vi "AK Namen.vi"(6 "Aktionen":T3, 7 "KV?":bool, 8 "EKFG Liste":string[](array[string]), 9 "AK Namen":string[](array[string]), 11 "Aktuelle Gasliste FT-IR":T1[](array[typedef])) -> (0 "EKFG Liste":string[](array[string]), 1 "AK Namen":string[](array[string]), 2 "Namen":string[](array[string]), 3 "AK Namen Liste":T2)   [LabVIEW 2020, in "AK-Schnittstelle.lvlib"]
uses:
  AK-Schnittstelle.lvlib
  AK Namen Aktionen.ctl
  AK Namen Listen.ctl
  Visualisierungs Elemente/String - Ausgabefeld.ctl
  SysLog/SysLog Interface.ctl
  Aktionen Gespeicherte Werte.ctl
  Allgemein/allgemeine Sub-VIs.lvlib
  Seiten/Gaszuordnung AO/Gaszuordnung AO.lvlib
  SysLog/SysLog.lvlib
  Aktion Array speichern.ctl
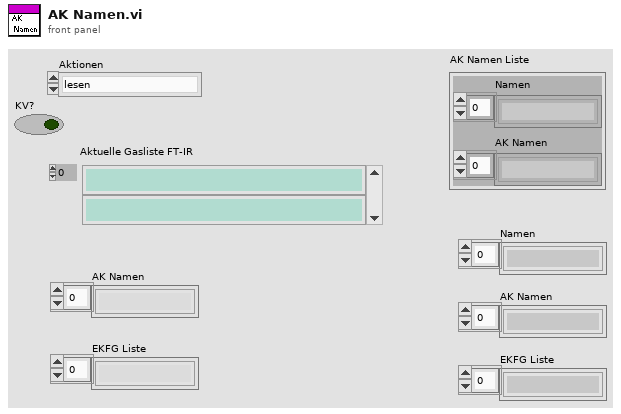
[diagram p1: front panel]
types:
  T1 = typedef "String - Ausgabefeld.ctl" = string
  T2 = typedef "AK-Schnittstelle.lvlib/AK Namen Listen.ctl" = cluster{"Namen":string[], "AK Namen":string[]}
  T3 = typedef "AK-Schnittstelle.lvlib/AK Namen Aktionen.ctl" = enum16{"lesen", "laden", "speichern Namen", "AK Namen", "Liste erstellen", "EKFG erstellen", "speichern EKFG", "EKFG schreiben", "Neuen Eintrag erzeugen"}
  T4 = typedef "SysLog.lvlib/SysLog Interface.ctl" = cluster{"FehlermeldungsCode":i32, "ErfolgsmeldungsCode":i32, "ParameterListenString":string, "Anzeige":bool, "SysLogIcon":enum16{"OK", "Warnung", "Fehler"}, "intern":bool}
  T5 = enum16{"open", "replace", "create", "open or create", "replace or create", "replace or create with confirmation"}
  T6 = typedef "AK-Schnittstelle.lvlib/Aktionen Gespeicherte Werte.ctl" = enum16{"lesen", "laden", "speichern", "Seriell", "TCP", "Diverse", "AKTIV", "AK-Namen"}
  T7 = typedef "AK-Schnittstelle.lvlib/Aktion Array speichern.ctl" = enum16{"AK Name ersetzen", "EKFG ersetzen", "Rezept fehler", "neues Rezept erstellen"}
  T8 = typedef "AK-Schnittstelle.lvlib/Diverse gespeicherte Werte.ctl" = cluster{"Kalibriergaseingang":i16, "SamplePoint":i16, "CalGas zu PNS":i16, "Gas-Reihenfolge":i16[], "Zeit 0-Gas":sgl, "Zeit CalGas":sgl, "AK Befehlssatz":T9}
  T9 = typedef "AK-Schnittstelle.lvlib/AK Befehlssatz.ctl" = enum16{"MEXA", "IAG v1.4", "AVL (Puma)", "PEUS"}
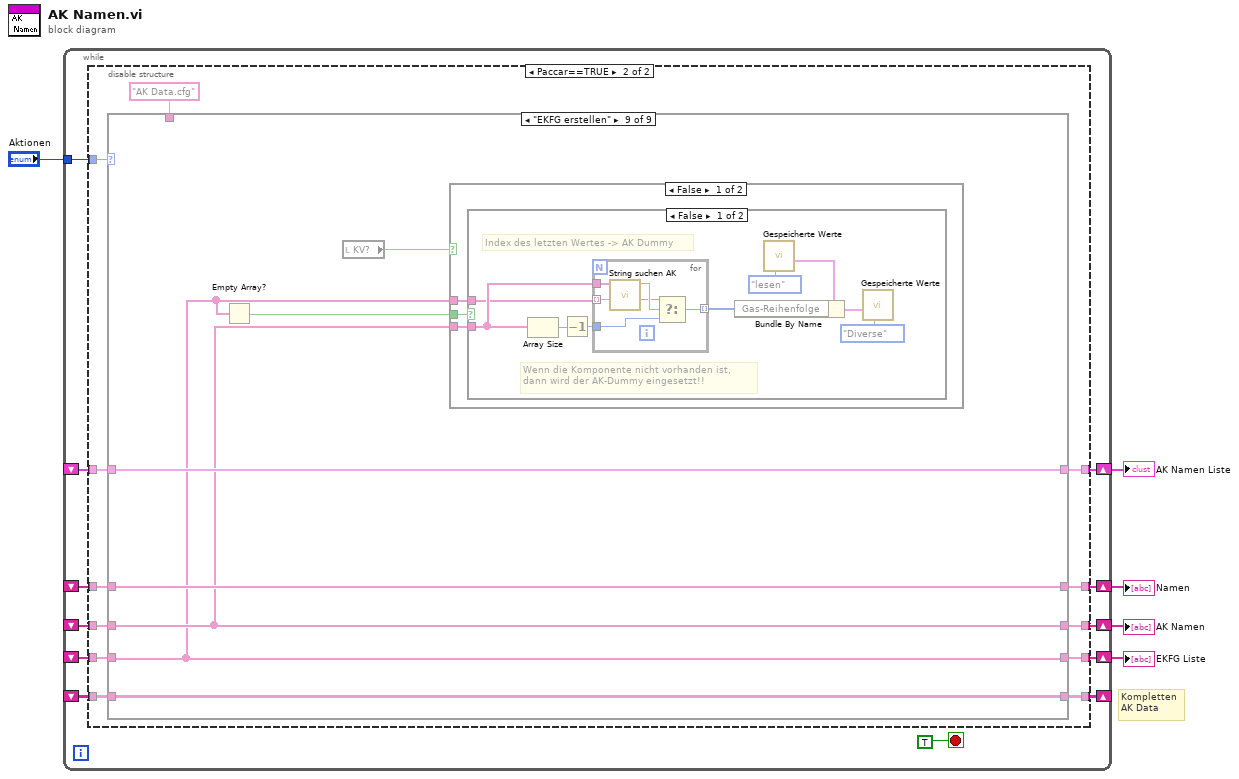
[diagram p0: block diagram]
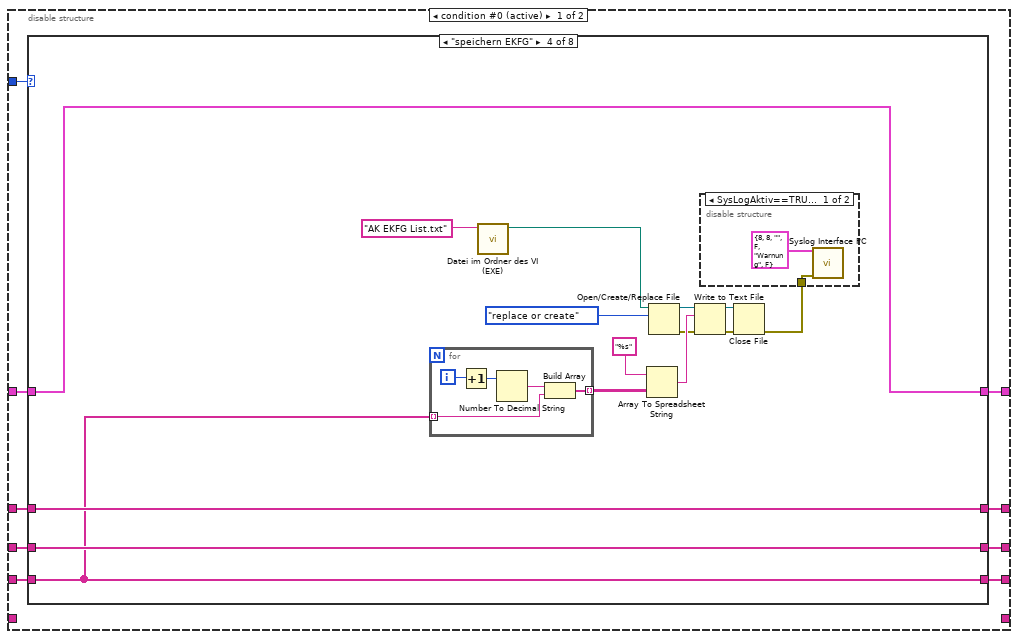
[diagram p2: hidden frame]
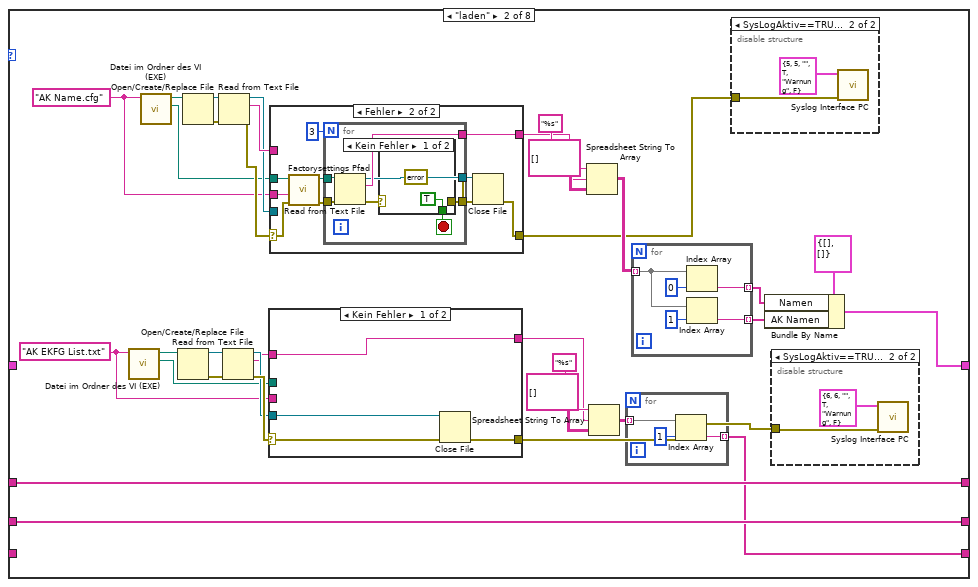
[diagram p4: hidden frame]
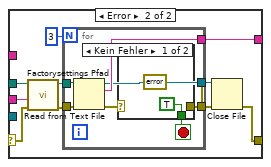
[diagram p7: hidden frame]
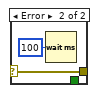
[diagram p8: hidden frame]
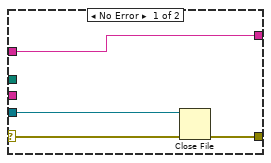
[diagram p9: hidden frame]
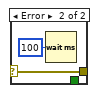
[diagram p10: hidden frame]
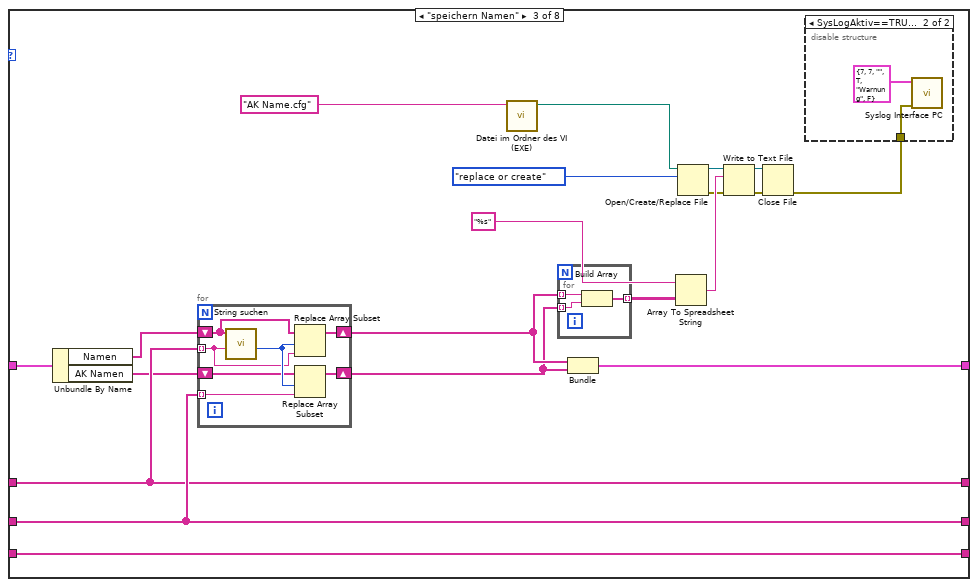
[diagram p11: hidden frame]
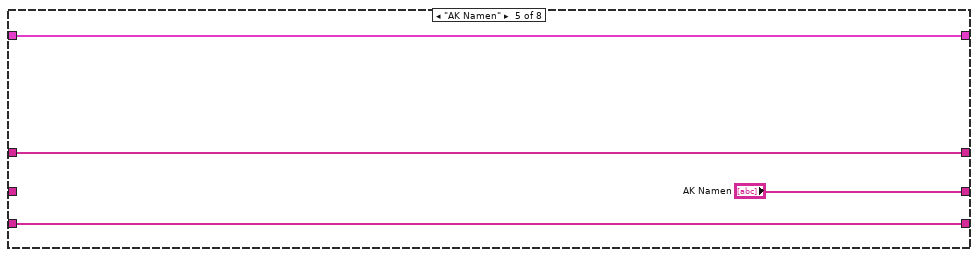
[diagram p14: hidden frame]
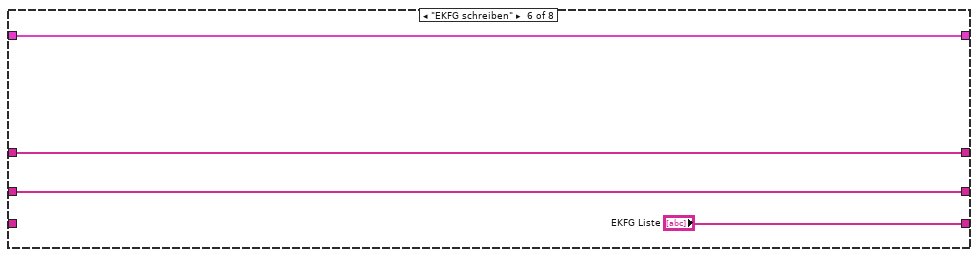
[diagram p15: hidden frame]
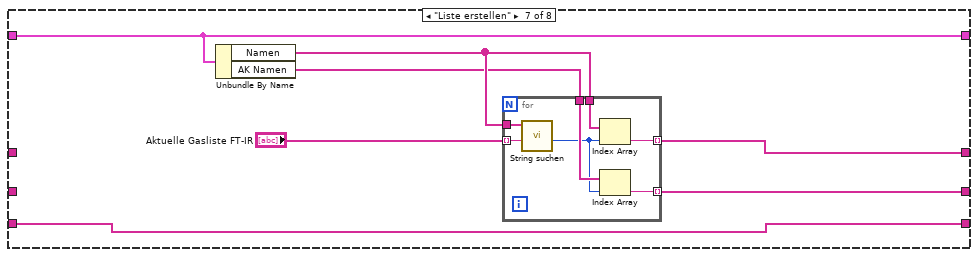
[diagram p16: hidden frame]
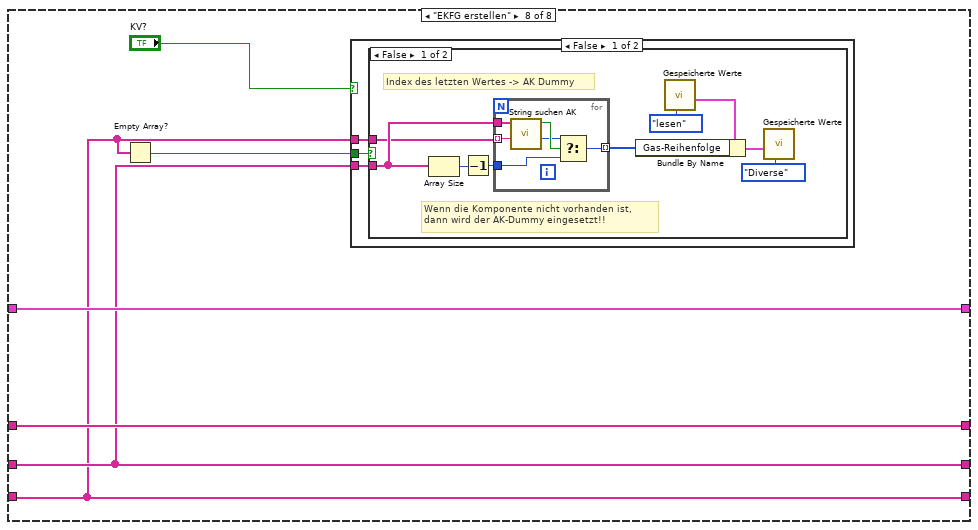
[diagram p17: hidden frame]
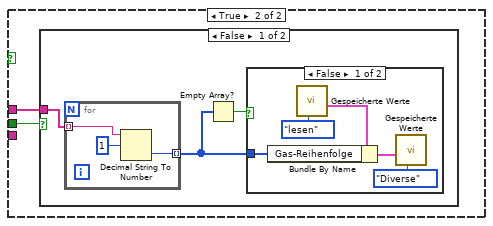
[diagram p19: hidden frame]
diagram:
  # "Kompletten\nAK Data"
  n1 = while {
    tunnel: "Aktionen" -> [w16]
    shift-right: [w15] -> w4
    shift-left: _ -> [w14]
    shift-right: [w12] -> w3
    shift-left: _ -> [w11]
    shift-right: [w13] -> w2
    shift-left: _ -> [w10]
    shift-right: [w9] -> w1
    shift-left: _ -> [w8]
    shift-right: [w7] -> _
    shift-left: _ -> [w6]
    stop <- TRUE stop-if-true
    n2 = disable-structure shown="Paccar==TRUE" {
      disable-tunnel: w16 -> [w26 w250]
      disable-tunnel: [w25 w249] -> w15
      disable-tunnel: w14 -> [w24 w248]
      disable-tunnel: [w23 w247] -> w13
      disable-tunnel: [w22 w246] -> w12
      disable-tunnel: w11 -> [w21 w245]
      disable-tunnel: w10 -> [w20 w244]
      disable-tunnel: [w19 w243] -> w9
      disable-tunnel: w8 -> [w18 w242]
      disable-tunnel: [_ w241] -> w7
      disable-tunnel: w6 -> [_ w240]
      frame condition #0 (active) {
        n3 = case shown="\"speichern EKFG\"" w26 {
          tunnel: [w30 w52 w143 w160 w182 w186 w194 w207] -> w25
          tunnel: w24 -> [w30 _ w145 w160 w182 w186 w194 w207]
          tunnel: [w28 w54 w144 w172 "AK Namen" w185 w191 w205] -> w23
          tunnel: [w29 w53 w142 w171 w183 w187 w190 w206] -> w22
          tunnel: w21 -> [w29 w53 w142 w171 w183 w187 _ w206]
          tunnel: w20 -> [w28 w54 w144 w172 _ w185 _ w205]
          tunnel: [w27 w45 w141 w170 w180 "EKFG Liste" w188 w204] -> w19
          tunnel: w18 -> [w27 _ w141 w170 w180 _ w188 w204]
          frame "lesen", Default {
          }
          frame "laden" {
            w34 = "AK EKFG List.txt" ("Dateiname")
            w40 = "AK Name.cfg" ("Dateiname")
            n4 = call "Datei im Ordner des VI (EXE).vi"("Dateiname"=w34) -> ("Ordner des Haupt-VIs"=w33:path, "Dateipfad im Ordner des Haupt-VIs"=w51:path)  [unwired: 8 in, 1 out]
            n5 = call "Datei im Ordner des VI (EXE).vi"("Dateiname"=w40) -> ("Ordner des Haupt-VIs"=w39:path, "Dateipfad im Ordner des Haupt-VIs"=w58:path)  [unwired: 8 in, 1 out]
            n6 = Open/Create/Replace File(file path (use dialog)=w51) -> (refnum out=w49:refnum<file>, error out=w50:errorcluster)  [unwired: 1 in, 5 out]
            n7 = Open/Create/Replace File(file path (use dialog)=w58) -> (refnum out=w60:refnum<file>, error out=w59:errorcluster)  [unwired: 1 in, 5 out]
            n8 = Read from Text File(file (use dialog)=w60, error in=w59) -> (refnum out=w41:refnum<file>, text=w44:string, error out=w42:errorcluster)  [unwired: 3 out]
            n9 = Read from Text File(file (use dialog)=w49, error in=w50) -> (refnum out=w36:refnum<file>, text=w35:string, error out=w37:errorcluster)  [unwired: 3 out]
            n10 = case shown="Kein Fehler" w37 {
              selector: w37 -> [w70 w73]
              tunnel: w33 -> [_ w74]
              tunnel: w35 -> [w71 _]
              tunnel: [w71 w80] -> w38
              tunnel: [w68 w78] -> w32
              tunnel: w36 -> [w69 _]
              tunnel: w34 -> [_ w72]
              frame No Error {
                n11 = Close File(refnum=w69, error in=w70) -> (error out=w68:errorcluster)  [unwired: 1 out]
              }
              frame Error {
                n12 = call "Factorysettings Pfad.vi"("error in (no error)"=w73, "Dateiname"=w72, "Ordner des Haupt-VIs"=w74) -> ("error out"=w75:errorcluster, "Pfad Factorysettings"=w76:path)  [unwired: 7 in]
                n13 = for {
                  N: 3 -> [_]
                  tunnel: w75 -> [w86]
                  tunnel: w76 -> [w85]
                  tunnel: [w84] -> w80
                  tunnel: [w83] -> w79
                  tunnel: [w82] -> w77
                  stop <- w87 stop-if-true
                  n14 = Read from Text File(file (use dialog)=w85, error in=w86) -> (refnum out=w82:refnum<file>, text=w84:string, error out=w88:errorcluster)  [unwired: 2 in, 1 out]
                  n15 = case shown="Kein Fehler" w88 {
                    selector: w88 -> [_ w91]
                    tunnel: [TRUE _] -> w87
                    tunnel: [errorcluster {"status"=FALSE, "code"=0, "source"=""} ("error IO") w91] -> w83
                    frame No Error {
                    }
                    frame Error {
                      n16 = Wait (ms)(milliseconds to wait=u32 100 ("Zu wartende ms")) -> ()  [unwired: 1 out]
                    }
                  }
                }
                n17 = Close File(refnum=w77, error in=w79) -> (error out=w78:errorcluster)  [unwired: 1 out]
              }
            }
            n18 = case shown="Fehler" w42 {
              selector: w42 -> [w95 w98]
              tunnel: w39 -> [_ w99]
              tunnel: w44 -> [w96 _]
              tunnel: [w96 w105] -> w43
              tunnel: [w93 w103] -> w31
              tunnel: w41 -> [w94 _]
              tunnel: w40 -> [_ w97]
              frame No Error {
                n19 = Close File(refnum=w94, error in=w95) -> (error out=w93:errorcluster)  [unwired: 1 out]
              }
              frame Error {
                n20 = call "Factorysettings Pfad.vi"("error in (no error)"=w98, "Dateiname"=w97, "Ordner des Haupt-VIs"=w99) -> ("error out"=w100:errorcluster, "Pfad Factorysettings"=w101:path)  [unwired: 7 in]
                n21 = for {
                  N: 3 -> [_]
                  tunnel: w100 -> [w111]
                  tunnel: w101 -> [w110]
                  tunnel: [w109] -> w105
                  tunnel: [w108] -> w104
                  tunnel: [w107] -> w102
                  stop <- w112 stop-if-true
                  n22 = Read from Text File(file (use dialog)=w110, error in=w111) -> (refnum out=w107:refnum<file>, text=w109:string, error out=w113:errorcluster)  [unwired: 2 in, 1 out]
                  n23 = case shown="Kein Fehler" w113 {
                    selector: w113 -> [_ w116]
                    tunnel: [TRUE _] -> w112
                    tunnel: [errorcluster {"status"=FALSE, "code"=0, "source"=""} ("error IO") w116] -> w108
                    frame No Error {
                    }
                    frame Error {
                      n24 = Wait (ms)(milliseconds to wait=u32 100 ("Zu wartende ms")) -> ()  [unwired: 1 out]
                    }
                  }
                }
                n25 = Close File(refnum=w102, error in=w104) -> (error out=w103:errorcluster)  [unwired: 1 out]
              }
            }
            n26 = Spreadsheet String To Array(format string="%s" ("Format-String"), spreadsheet string=w43, array type (2D Dbl)=string[][] []) -> (array=w63:string[][])  [unwired: 1 out]
            n27 = Spreadsheet String To Array(format string="%s" ("Format-String"), spreadsheet string=w38, array type (2D Dbl)=string[][] []) -> (array=w46:string[][])  [unwired: 1 out]
            n28 = for {
              tunnel: w46 -> [w118] mode=indexing
              tunnel: [w119] -> w45 mode=indexing
              n29 = Index Array(array=w118, index=1 ("Index")) -> (element=w119:string)
            }
            n30 = for {
              tunnel: w63 -> [w121] mode=indexing
              tunnel: [w123] -> w55 mode=indexing
              tunnel: [w122] -> w56 mode=indexing
              n31 = Index Array(array=w121, index=0 ("Index")) -> (element=w123:string)
              n32 = Index Array(array=w121, index=1 ("Index")) -> (element=w122:string)
            }
            n33 = disable-structure shown="SysLogAktiv==TRUE" {
              disable-tunnel: w31 -> [_ w65]
              frame condition #0 {
              }
              frame condition #1 (active) {
                n34 = call "Syslog Interface PC.vi"("Fehler (in)"=w65, "Cluster (in)"=T4 {"FehlermeldungsCode"=5, "ErfolgsmeldungsCode"=5, "ParameterListenString"="", "Anzeige"=TRUE, "SysLogIcon"=enum."Warnung", "intern"=FALSE}) -> ()  [unwired: 9 in, 1 out]
              }
            }
            n35 = Bundle By Name(cluster=T2 {"Namen"=[], "AK Namen"=[]} ("Polynome"), "Namen"=w55, "AK Namen"=w56) -> (w52:T2)
            n36 = disable-structure shown="SysLogAktiv==TRUE" {
              disable-tunnel: w32 -> [_ w67]
              frame condition #0 {
              }
              frame condition #1 (active) {
                n37 = call "Syslog Interface PC.vi"("Fehler (in)"=w67, "Cluster (in)"=T4 {"FehlermeldungsCode"=6, "ErfolgsmeldungsCode"=6, "ParameterListenString"="", "Anzeige"=TRUE, "SysLogIcon"=enum."Warnung", "intern"=FALSE}) -> ()  [unwired: 9 in, 1 out]
              }
            }
          }
          frame "speichern Namen" {
            n38 = Unbundle By Name(w145) -> ("Namen"=w129:string[], "AK Namen"=w128:string[])
            n39 = for {
              tunnel: w142 -> [w154] mode=indexing
              tunnel: w144 -> [w151] mode=indexing
              shift-right: [w156] -> w131
              shift-left: w129 -> [w153]
              shift-right: [w155] -> w130
              shift-left: w128 -> [w152]
              n40 = call "String suchen.vi"("Gasname"=w154, "Such-Namen"=w153) -> ("Index"=w157:i32)  [unwired: 8 in, 1 out]
              n41 = Replace Array Subset(array=w153, new element=w154, index=w157) -> (w156:string[])
              n42 = Replace Array Subset(array=w152, new element=w151, index=w157) -> (w155:string[])
            }
            n43 = call "Datei im Ordner des VI (EXE).vi"("Dateiname"="AK Name.cfg") -> ("Dateipfad im Ordner des Haupt-VIs"=w133:path)  [unwired: 8 in, 2 out]
            n44 = for {
              tunnel: w131 -> [w148] mode=indexing
              tunnel: [w150] -> w132 mode=indexing
              tunnel: w130 -> [w149] mode=indexing
              n45 = Build Array(w148, w149) -> (w150:string[])
            }
            n46 = Bundle("Namen"=w131, "AK Namen"=w130) -> (w143:cluster{"Namen":string[], "AK Namen":string[]})  [unwired: 1 in]
            n47 = Array To Spreadsheet String(array=w132, 3:"%s" ("Format-String")) -> (spreadsheet string=w138:string)  [unwired: 1 out]
            n48 = Open/Create/Replace File(file path (use dialog)=w133, operation (0:open)=T5."replace or create" ("Operation (0:Öffnen)")) -> (refnum out=w139:refnum<file>, error out=w135:errorcluster)  [unwired: 1 in, 4 out]
            n49 = Write to Text File(file (use dialog)=w139, text=w138, error in=w135) -> (refnum out=w136:refnum<file>, error out=w137:errorcluster)  [unwired: 2 out]
            n50 = Close File(refnum=w136, error in=w137) -> (error out=w127:errorcluster)  [unwired: 1 out]
            n51 = disable-structure shown="SysLogAktiv==TRUE" {
              disable-tunnel: w127 -> [_ w147]
              frame condition #0 {
              }
              frame condition #1 (active) {
                n52 = call "Syslog Interface PC.vi"("Fehler (in)"=w147, "Cluster (in)"=T4 {"FehlermeldungsCode"=7, "ErfolgsmeldungsCode"=7, "ParameterListenString"="", "Anzeige"=TRUE, "SysLogIcon"=enum."Warnung", "intern"=FALSE}) -> ()  [unwired: 9 in, 1 out]
              }
            }
          }
          frame "speichern EKFG" {
            n53 = for {
              tunnel: w170 -> [w176] mode=indexing
              tunnel: [w175] -> w161 mode=indexing
              i -> [w179]
              n54 = Increment(x=w179) -> (x+1=w178:i32)
              n55 = Number To Decimal String(number=w178) -> (decimal integer string=w177:string)  [unwired: 1 in]
              n56 = Build Array(w177, w176) -> (w175:string[])
            }
            n57 = call "Datei im Ordner des VI (EXE).vi"("Dateiname"="AK EKFG List.txt") -> ("Dateipfad im Ordner des Haupt-VIs"=w162:path)  [unwired: 8 in, 2 out]
            n58 = Array To Spreadsheet String(array=w161, 3:"%s" ("Format-String")) -> (spreadsheet string=w167:string)  [unwired: 1 out]
            n59 = Open/Create/Replace File(file path (use dialog)=w162, operation (0:open)=T5."replace or create" ("Operation (0:Öffnen)")) -> (refnum out=w168:refnum<file>, error out=w164:errorcluster)  [unwired: 1 in, 4 out]
            n60 = Write to Text File(file (use dialog)=w168, text=w167, error in=w164) -> (refnum out=w165:refnum<file>, error out=w166:errorcluster)  [unwired: 2 out]
            n61 = Close File(refnum=w165, error in=w166) -> (error out=w158:errorcluster)  [unwired: 1 out]
            n62 = disable-structure shown="SysLogAktiv==TRUE" {
              disable-tunnel: w158 -> [w174 _]
              frame condition #0 (active) {
                n63 = call "Syslog Interface PC.vi"("Fehler (in)"=w174, "Cluster (in)"=T4 {"FehlermeldungsCode"=8, "ErfolgsmeldungsCode"=8, "ParameterListenString"="", "Anzeige"=FALSE, "SysLogIcon"=enum."Warnung", "intern"=FALSE}) -> ()  [unwired: 9 in, 1 out]
              }
              frame condition #1 {
              }
            }
          }
          frame "AK Namen" {
          }
          frame "EKFG schreiben" {
          }
          frame "Liste erstellen" {
            n64 = Unbundle By Name(w194) -> ("Namen"=w193:string[], "AK Namen"=w192:string[])
            n65 = for {
              tunnel: "Aktuelle Gasliste FT-IR" -> [w201] mode=indexing
              tunnel: w193 -> [w200]
              tunnel: w193 -> [w199]
              tunnel: w192 -> [w198]
              tunnel: [w197] -> w190 mode=indexing
              tunnel: [w196] -> w191 mode=indexing
              n66 = call "String suchen.vi"("Gasname"=w201, "Such-Namen"=w200) -> ("Index"=w195:i32)  [unwired: 8 in, 1 out]
              n67 = Index Array(array=w199, index=w195) -> (element=w197:string)
              n68 = Index Array(array=w198, index=w195) -> (element=w196:string)
            }
          }
          frame "EKFG erstellen" {
            n69 = Empty Array?(array=w204) -> (empty?=w203:bool)
            n70 = case shown="False" "KV?" {
              tunnel: w205 -> [w210 _]
              tunnel: w204 -> [w209 w226]
              tunnel: w203 -> [w208 w227]
              frame False {
                n71 = case shown="False" w208 {
                  tunnel: w210 -> [w213 _]
                  tunnel: w209 -> [w211 _]
                  frame False {
                    # "Wenn die Komponente nicht vorhanden ist, \ndann wird der AK-Dummy eingesetzt!!"
                    # "Index des letzten Wertes -> AK Dummy"
                    n72 = Array Size(array=w213) -> (size(s)=w215:i32)
                    n73 = Decrement(x=w215) -> (x-1=w212:i32)
                    n74 = for {
                      tunnel: w211 -> [w224] mode=indexing
                      tunnel: [w221] -> w214 mode=indexing
                      tunnel: w213 -> [w225]
                      tunnel: w212 -> [w220]
                      n75 = call "String suchen AK.vi"("gesucht"=w224, "Namen"=w225) -> ("Index"=w222:i32, "Gefunden?"=w223:bool)  [unwired: 8 in]
                      n76 = Select(t=w222, s=w223, f=w220) -> (s? t:f=w221:i32)
                    }
                    n77 = call "Gespeicherte Werte.vi"("Aktionen"=Aktionen_Gespeicherte_Werte."lesen") -> ("Diverse Werte"=w218:T8)  [unwired: 6 in, 4 out]
                    n78 = Bundle By Name(cluster=w218, "Gas-Reihenfolge"=w214) -> (w219:T8)
                    n79 = call "Gespeicherte Werte.vi"("Aktionen"=Aktionen_Gespeicherte_Werte."Diverse", "Diverse Werte"=w219) -> ()  [unwired: 5 in, 5 out]
                  }
                  frame True {
                  }
                }
              }
              frame True {
                n80 = case shown="False" w227 {
                  tunnel: w226 -> [w228 _]
                  frame False {
                    n81 = for {
                      tunnel: w228 -> [w237] mode=indexing
                      tunnel: [w236] -> w229 mode=indexing
                      n82 = Decimal String To Number(string=w237, offset=1 ("Offset")) -> (number=w236:i32)  [unwired: 1 in, 1 out]
                    }
                    n83 = Empty Array?(array=w229) -> (empty?=w230:bool)
                    n84 = case shown="False" w230 {
                      tunnel: w229 -> [w231 _]
                      frame False {
                        n85 = call "Gespeicherte Werte.vi"("Aktionen"=Aktionen_Gespeicherte_Werte."lesen") -> ("Diverse Werte"=w234:T8)  [unwired: 6 in, 4 out]
                        n86 = Bundle By Name(cluster=w234, "Gas-Reihenfolge"=w231) -> (w235:T8)
                        n87 = call "Gespeicherte Werte.vi"("Aktionen"=Aktionen_Gespeicherte_Werte."Diverse", "Diverse Werte"=w235) -> ()  [unwired: 5 in, 5 out]
                      }
                      frame True {
                      }
                    }
                  }
                  frame True {
                  }
                }
              }
            }
          }
        }
      }
      frame condition #1 {
        n88 = case shown="\"EKFG erstellen\"" w250 {
          tunnel: [w255 w271 w336 w377 w403 w425 w430 w439 w453] -> w249
          tunnel: w248 -> [w255 _ w338 w379 w403 w425 w430 w439 w453]
          tunnel: [w253 w273 w337 w378 w414 w423 w429 w436 w451] -> w247
          tunnel: [w254 w272 w335 w376 w413 w426 w431 w435 w452] -> w246
          tunnel: w245 -> [w254 w272 w335 w376 w413 w426 w431 _ w452]
          tunnel: w244 -> [w253 w273 w337 w378 w414 _ w429 _ w451]
          tunnel: [w252 w270 w316 w357 w412 w424 w428 w434 w450] -> w243
          tunnel: w242 -> [w252 _ w316 w357 w412 w424 _ w434 w450]
          tunnel: [w251 w257 w317 w358 w398 w422 w427 w432 w448] -> w241
          tunnel: w240 -> [w251 _ w318 w359 w400 w422 w427 w432 w448]
          tunnel: "AK Data.cfg" ("Dateiname") -> [_ w256 w320 w361 w401 _ _ _ _]
          frame "lesen", Default {
          }
          frame "laden" {
            n89 = call "Datei im Ordner des VI (EXE).vi"("Dateiname"=w256) -> ("Ordner des Haupt-VIs"=w266:path, "Dateipfad im Ordner des Haupt-VIs"=w277:path)  [unwired: 8 in, 1 out]
            n90 = Open/Create/Replace File(file path (use dialog)=w277) -> (refnum out=w279:refnum<file>, error out=w278:errorcluster)  [unwired: 1 in, 5 out]
            n91 = Read from Text File(file (use dialog)=w279, error in=w278) -> (refnum out=w267:refnum<file>, text=w269:string, error out=w268:errorcluster)  [unwired: 3 out]
            n92 = case shown="Fehler" w268 {
              selector: w268 -> [w284 w287]
              tunnel: w266 -> [_ w288]
              tunnel: w269 -> [w285 _]
              tunnel: [w285 w294] -> w258
              tunnel: [w282 w292] -> w265
              tunnel: w267 -> [w283 _]
              tunnel: w256 -> [_ w286]
              frame No Error {
                n93 = Close File(refnum=w283, error in=w284) -> (error out=w282:errorcluster)  [unwired: 1 out]
              }
              frame Error {
                n94 = call "Factorysettings Pfad.vi"("error in (no error)"=w287, "Dateiname"=w286, "Ordner des Haupt-VIs"=w288) -> ("error out"=w289:errorcluster, "Pfad Factorysettings"=w290:path)  [unwired: 7 in]
                n95 = for {
                  N: 3 -> [_]
                  tunnel: w289 -> [w300]
                  tunnel: w290 -> [w299]
                  tunnel: [w298] -> w294
                  tunnel: [w297] -> w293
                  tunnel: [w296] -> w291
                  stop <- w301 stop-if-true
                  n96 = Read from Text File(file (use dialog)=w299, error in=w300) -> (refnum out=w296:refnum<file>, text=w298:string, error out=w302:errorcluster)  [unwired: 2 in, 1 out]
                  n97 = case shown="Kein Fehler" w302 {
                    selector: w302 -> [_ w305]
                    tunnel: [TRUE _] -> w301
                    tunnel: [errorcluster {"status"=FALSE, "code"=0, "source"=""} ("error IO") w305] -> w297
                    frame No Error {
                    }
                    frame Error {
                      n98 = Wait (ms)(milliseconds to wait=u32 100 ("Zu wartende ms")) -> ()  [unwired: 1 out]
                    }
                  }
                }
                n99 = Close File(refnum=w291, error in=w293) -> (error out=w292:errorcluster)  [unwired: 1 out]
              }
            }
            n100 = call "Recipe array ausgeben.vi"("Komplette Datei"=w258) -> ("Recipe Teil"=w263:string[][], "error out"=w264:errorcluster)  [unwired: 11 in, 2 out]
            n101 = Spreadsheet String To Array(format string="%s" ("Format-String"), spreadsheet string=w258, array type (2D Dbl)=string[][] []) -> (array=w257:string[][])  [unwired: 1 in]
            n102 = disable-structure shown="SysLogAktiv==TRUE" {
              disable-tunnel: w265 -> [_ w281]
              frame condition #0 {
              }
              frame condition #1 (active) {
                n103 = call "Syslog Interface PC.vi"("Fehler (in)"=w281, "Cluster (in)"=T4 {"FehlermeldungsCode"=5, "ErfolgsmeldungsCode"=5, "ParameterListenString"="", "Anzeige"=TRUE, "SysLogIcon"=enum."Warnung", "intern"=FALSE}) -> ()  [unwired: 9 in, 1 out]
              }
            }
            n104 = call "Split AK Name und EKFG.vi"("Recipe Teil"=w263, "error in (no error)"=w264) -> ("AK Name"=w262:string[][], "EKFG"=w261:string[][])  [unwired: 9 in, 3 out]
            n105 = for {
              tunnel: w261 -> [w307] mode=indexing
              tunnel: [w308] -> w270 mode=indexing
              n106 = Index Array(array=w307, index=1 ("Index")) -> (element=w308:string)
            }
            n107 = for {
              tunnel: w262 -> [w310] mode=indexing
              tunnel: [w312] -> w274 mode=indexing
              tunnel: [w311] -> w275 mode=indexing
              n108 = Index Array(array=w310, index=0 ("Index")) -> (element=w312:string)
              n109 = Index Array(array=w310, index=1 ("Index")) -> (element=w311:string)
            }
            n110 = Bundle By Name(cluster=T2 {"Namen"=[], "AK Namen"=[]} ("Polynome"), "Namen"=w274, "AK Namen"=w275) -> (w271:T2)
          }
          frame "speichern Namen" {
            n111 = Unbundle By Name(w338) -> ("Namen"=w326:string[], "AK Namen"=w325:string[])
            n112 = for {
              tunnel: w316 -> [w340] mode=indexing
              tunnel: [w339] -> w315 mode=indexing
              i -> [w343]
              n113 = Increment(x=w343) -> (x+1=w342:i32)
              n114 = Number To Decimal String(number=w342) -> (decimal integer string=w341:string)  [unwired: 1 in]
              n115 = Build Array(w341, w340) -> (w339:string[])
            }
            n116 = for {
              tunnel: w335 -> [w352] mode=indexing
              tunnel: w337 -> [w349] mode=indexing
              shift-right: [w354] -> w328
              shift-left: w326 -> [w351]
              shift-right: [w353] -> w327
              shift-left: w325 -> [w350]
              n117 = call "String suchen.vi"("Gasname"=w352, "Such-Namen"=w351) -> ("Index"=w355:i32)  [unwired: 8 in, 1 out]
              n118 = Replace Array Subset(array=w351, new element=w352, index=w355) -> (w354:string[])
              n119 = Replace Array Subset(array=w350, new element=w349, index=w355) -> (w353:string[])
            }
            n120 = for {
              tunnel: w328 -> [w346] mode=indexing
              tunnel: [w348] -> w319 mode=indexing
              tunnel: w327 -> [w347] mode=indexing
              n121 = Build Array(w346, w347) -> (w348:string[])
            }
            n122 = call "Teil Array speichern.vi"("Komplette Datei"=w318, "AK NAME Teil"=w319, "EKFG Teil"=w315, "Aktion"=Aktion_Array_speichern."AK Name ersetzen") -> ("Komplette Datei"=w317:string[][])  [unwired: 8 in, 3 out]
            n123 = Bundle("Namen"=w328, "AK Namen"=w327) -> (w336:cluster{"Namen":string[], "AK Namen":string[]})  [unwired: 1 in]
            n124 = call "Datei im Ordner des VI (EXE).vi"("Dateiname"=w320) -> ("Dateipfad im Ordner des Haupt-VIs"=w329:path)  [unwired: 8 in, 2 out]
            n125 = Array To Spreadsheet String(array=w317, 3:"%s" ("Format-String")) -> (spreadsheet string=w322:string)  [unwired: 1 in]
            n126 = Open/Create/Replace File(file path (use dialog)=w329, operation (0:open)=T5."replace or create" ("Operation (0:Öffnen)")) -> (refnum out=w334:refnum<file>, error out=w331:errorcluster)  [unwired: 1 in, 4 out]
            n127 = Write to Text File(file (use dialog)=w334, text=w322, error in=w331) -> (refnum out=w332:refnum<file>, error out=w333:errorcluster)  [unwired: 2 out]
            n128 = Close File(refnum=w332, error in=w333) -> (error out=w324:errorcluster)  [unwired: 1 out]
            n129 = disable-structure shown="SysLogAktiv==TRUE" {
              disable-tunnel: w324 -> [_ w345]
              frame condition #0 {
              }
              frame condition #1 (active) {
                n130 = call "Syslog Interface PC.vi"("Fehler (in)"=w345, "Cluster (in)"=T4 {"FehlermeldungsCode"=7, "ErfolgsmeldungsCode"=7, "ParameterListenString"="", "Anzeige"=TRUE, "SysLogIcon"=enum."Warnung", "intern"=FALSE}) -> ()  [unwired: 9 in, 1 out]
              }
            }
          }
          frame "Neuen Eintrag erzeugen" {
            n131 = Unbundle By Name(w379) -> ("Namen"=w367:string[], "AK Namen"=w366:string[])
            n132 = for {
              tunnel: w376 -> [w393] mode=indexing
              tunnel: w378 -> [w390] mode=indexing
              shift-right: [w395] -> w369
              shift-left: w367 -> [w392]
              shift-right: [w394] -> w368
              shift-left: w366 -> [w391]
              n133 = call "String suchen.vi"("Gasname"=w393, "Such-Namen"=w392) -> ("Index"=w396:i32)  [unwired: 8 in, 1 out]
              n134 = Replace Array Subset(array=w392, new element=w393, index=w396) -> (w395:string[])
              n135 = Replace Array Subset(array=w391, new element=w390, index=w396) -> (w394:string[])
            }
            n136 = for {
              tunnel: w357 -> [w381] mode=indexing
              tunnel: [w380] -> w356 mode=indexing
              i -> [w384]
              n137 = Increment(x=w384) -> (x+1=w383:i32)
              n138 = Number To Decimal String(number=w383) -> (decimal integer string=w382:string)  [unwired: 1 in]
              n139 = Build Array(w382, w381) -> (w380:string[])
            }
            n140 = for {
              tunnel: w369 -> [w387] mode=indexing
              tunnel: [w389] -> w360 mode=indexing
              tunnel: w368 -> [w388] mode=indexing
              n141 = Build Array(w387, w388) -> (w389:string[])
            }
            n142 = call "Teil Array speichern.vi"("Komplette Datei"=w359, "AK NAME Teil"=w360, "EKFG Teil"=w356, "Aktion"=Aktion_Array_speichern."neues Rezept erstellen") -> ("Komplette Datei"=w358:string[][])  [unwired: 8 in, 3 out]
            n143 = Bundle("Namen"=w369, "AK Namen"=w368) -> (w377:cluster{"Namen":string[], "AK Namen":string[]})  [unwired: 1 in]
            n144 = call "Datei im Ordner des VI (EXE).vi"("Dateiname"=w361) -> ("Dateipfad im Ordner des Haupt-VIs"=w370:path)  [unwired: 8 in, 2 out]
            n145 = Array To Spreadsheet String(array=w358, 3:"%s" ("Format-String")) -> (spreadsheet string=w363:string)  [unwired: 1 in]
            n146 = Open/Create/Replace File(file path (use dialog)=w370, operation (0:open)=T5."replace or create" ("Operation (0:Öffnen)")) -> (refnum out=w375:refnum<file>, error out=w372:errorcluster)  [unwired: 1 in, 4 out]
            n147 = Write to Text File(file (use dialog)=w375, text=w363, error in=w372) -> (refnum out=w373:refnum<file>, error out=w374:errorcluster)  [unwired: 2 out]
            n148 = Close File(refnum=w373, error in=w374) -> (error out=w365:errorcluster)  [unwired: 1 out]
            n149 = disable-structure shown="SysLogAktiv==TRUE" {
              disable-tunnel: w365 -> [_ w386]
              frame condition #0 {
              }
              frame condition #1 (active) {
                n150 = call "Syslog Interface PC.vi"("Fehler (in)"=w386, "Cluster (in)"=T4 {"FehlermeldungsCode"=7, "ErfolgsmeldungsCode"=7, "ParameterListenString"="", "Anzeige"=TRUE, "SysLogIcon"=enum."Warnung", "intern"=FALSE}) -> ()  [unwired: 9 in, 1 out]
              }
            }
          }
          frame "speichern EKFG" {
            n151 = for {
              tunnel: w412 -> [w418] mode=indexing
              tunnel: [w417] -> w399 mode=indexing
              i -> [w421]
              n152 = Increment(x=w421) -> (x+1=w420:i32)
              n153 = Number To Decimal String(number=w420) -> (decimal integer string=w419:string)  [unwired: 1 in]
              n154 = Build Array(w419, w418) -> (w417:string[])
            }
            n155 = call "Teil Array speichern.vi"("Komplette Datei"=w400, "EKFG Teil"=w399, "Aktion"=Aktion_Array_speichern."EKFG ersetzen") -> ("Komplette Datei"=w398:string[][])  [unwired: 9 in, 3 out]
            n156 = call "Datei im Ordner des VI (EXE).vi"("Dateiname"=w401) -> ("Dateipfad im Ordner des Haupt-VIs"=w404:path)  [unwired: 8 in, 2 out]
            n157 = Array To Spreadsheet String(array=w398, 3:"%s" ("Format-String")) -> (spreadsheet string=w409:string)  [unwired: 1 out]
            n158 = Open/Create/Replace File(file path (use dialog)=w404, operation (0:open)=T5."replace or create" ("Operation (0:Öffnen)")) -> (refnum out=w410:refnum<file>, error out=w406:errorcluster)  [unwired: 1 in, 4 out]
            n159 = Write to Text File(file (use dialog)=w410, text=w409, error in=w406) -> (refnum out=w407:refnum<file>, error out=w408:errorcluster)  [unwired: 2 out]
            n160 = Close File(refnum=w407, error in=w408) -> (error out=w402:errorcluster)  [unwired: 1 out]
            n161 = disable-structure shown="SysLogAktiv==TRUE" {
              disable-tunnel: w402 -> [w416 _]
              frame condition #0 (active) {
                n162 = call "Syslog Interface PC.vi"("Fehler (in)"=w416, "Cluster (in)"=T4 {"FehlermeldungsCode"=8, "ErfolgsmeldungsCode"=8, "ParameterListenString"="", "Anzeige"=FALSE, "SysLogIcon"=enum."Warnung", "intern"=FALSE}) -> ()  [unwired: 9 in, 1 out]
              }
              frame condition #1 {
              }
            }
          }
          frame "AK Namen" {
            n163 = local read "AK Namen"() -> (w423:string[])
          }
          frame "EKFG schreiben" {
            n164 = local read "EKFG Liste"() -> (w428:string[])
          }
          frame "Liste erstellen" {
            n165 = Unbundle By Name(w439) -> ("Namen"=w438:string[], "AK Namen"=w437:string[])
            n166 = local read "Aktuelle Gasliste FT-IR"() -> (w433:T1[])
            n167 = for {
              tunnel: w433 -> [w446] mode=indexing
              tunnel: w438 -> [w445]
              tunnel: w438 -> [w444]
              tunnel: w437 -> [w443]
              tunnel: [w442] -> w435 mode=indexing
              tunnel: [w441] -> w436 mode=indexing
              n168 = call "String suchen.vi"("Gasname"=w446, "Such-Namen"=w445) -> ("Index"=w440:i32)  [unwired: 8 in, 1 out]
              n169 = Index Array(array=w444, index=w440) -> (element=w442:string)
              n170 = Index Array(array=w443, index=w440) -> (element=w441:string)
            }
          }
          frame "EKFG erstellen" {
            n171 = Empty Array?(array=w450) -> (empty?=w449:bool)
            n172 = local read "KV?"() -> (w447:bool)
            n173 = case shown="False" w447 {
              tunnel: w451 -> [w456 _]
              tunnel: w450 -> [w455 w472]
              tunnel: w449 -> [w454 w473]
              frame False {
                n174 = case shown="False" w454 {
                  tunnel: w456 -> [w459 _]
                  tunnel: w455 -> [w457 _]
                  frame False {
                    # "Wenn die Komponente nicht vorhanden ist, \ndann wird der AK-Dummy eingesetzt!!"
                    # "Index des letzten Wertes -> AK Dummy"
                    n175 = Array Size(array=w459) -> (size(s)=w461:i32)
                    n176 = Decrement(x=w461) -> (x-1=w458:i32)
                    n177 = for {
                      tunnel: w457 -> [w470] mode=indexing
                      tunnel: [w467] -> w460 mode=indexing
                      tunnel: w459 -> [w471]
                      tunnel: w458 -> [w466]
                      n178 = call "String suchen AK.vi"("gesucht"=w470, "Namen"=w471) -> ("Index"=w468:i32, "Gefunden?"=w469:bool)  [unwired: 8 in]
                      n179 = Select(t=w468, s=w469, f=w466) -> (s? t:f=w467:i32)
                    }
                    n180 = call "Gespeicherte Werte.vi"("Aktionen"=Aktionen_Gespeicherte_Werte."lesen") -> ("Diverse Werte"=w464:T8)  [unwired: 6 in, 4 out]
                    n181 = Bundle By Name(cluster=w464, "Gas-Reihenfolge"=w460) -> (w465:T8)
                    n182 = call "Gespeicherte Werte.vi"("Aktionen"=Aktionen_Gespeicherte_Werte."Diverse", "Diverse Werte"=w465) -> ()  [unwired: 5 in, 5 out]
                  }
                  frame True {
                  }
                }
              }
              frame True {
                n183 = case shown="False" w473 {
                  tunnel: w472 -> [w474 _]
                  frame False {
                    n184 = for {
                      tunnel: w474 -> [w483] mode=indexing
                      tunnel: [w482] -> w475 mode=indexing
                      n185 = Decimal String To Number(string=w483, offset=1 ("Offset")) -> (number=w482:i32)  [unwired: 1 in, 1 out]
                    }
                    n186 = Empty Array?(array=w475) -> (empty?=w476:bool)
                    n187 = case shown="False" w476 {
                      tunnel: w475 -> [w477 _]
                      frame False {
                        n188 = call "Gespeicherte Werte.vi"("Aktionen"=Aktionen_Gespeicherte_Werte."lesen") -> ("Diverse Werte"=w480:T8)  [unwired: 6 in, 4 out]
                        n189 = Bundle By Name(cluster=w480, "Gas-Reihenfolge"=w477) -> (w481:T8)
                        n190 = call "Gespeicherte Werte.vi"("Aktionen"=Aktionen_Gespeicherte_Werte."Diverse", "Diverse Werte"=w481) -> ()  [unwired: 5 in, 5 out]
                      }
                      frame True {
                      }
                    }
                  }
                  frame True {
                  }
                }
              }
            }
          }
        }
      }
    }
  }
  "AK Namen Liste" <- w4
  "Namen" <- w3
  "AK Namen" <- w2
  "EKFG Liste" <- w1
